vi "2014 Robot Global Data.vi"() -> ()   [LabVIEW 2013]
doc: "This global VI can contain as many global variables as you need. Place a control on the panel, give it a good name. To read or write to it from a VI, drag the icon to the diagram of that VI. You can also drag from the project. Click on the node to change which global you access. You shouldn't have multiple locations writing to a global or it will cause a race-condition."
uses:
  <vilib>/Rock Robotics/WPI/DriverStation/WPI_DriverStationRobotMode2.ctl
  <vilib>/Rock Robotics/WPI/Camera/WPI_CameraImageSize.ctl
panel:
  in  "Tab Control":T1(tab)=enum."I/O Definitions"
  in  "Enable Temp 16":bool
  in  "Enable Temp 15":bool
  in  "Enable Temp 14":bool
  in  "Enable Ejector":bool=TRUE
  in  "Enable Illuminators":bool
  in  "Enable PWM Wheels":bool
  in  "Enable CAN Voltage Wheels":bool=TRUE
  in  "Enable CAN Speed Wheels":bool
  in  "Enable Compressor":bool=TRUE
  in  "Enable Vision":bool
  in  "Enable I2C Accelerometer":bool=TRUE
  in  "Enable Gyro Temp":bool=TRUE
  in  "Enable Gyro":bool=TRUE
  in  "Enable Shooter Tilt":bool=TRUE
  in  "Enable Pickup Rollers":bool=TRUE
  in  "Enable Shooter Wheels":bool=TRUE
  in  "Robot Mode":T2=enum."Finish"
  in  "LED toggle rate (ms)":u32=250
  in  "image size":T3=enum."320x240"
  in  "Accelerometer Gain":dbl=1.0
  in  "Gyro Gain\n(VoltsPerDegree/Second)":dbl=0.007
  out "Gyro Temp":dbl
  out "Gyro Angle":dbl=2.5745306100192002
  out "Gyro Rate":dbl=-0.02367994921875
  out "Battery Voltage":dbl=12.69887799264
  out "X-Acceleration":i16
  out "Y-Acceleration":i16
  out "Z-Acceleration":i16
  in  "Drive Wheel Scale":dbl=1.0
  in  "Wheel Kd":dbl
  in  "Wheel Ki":dbl=0.004
  in  "Wheel Kp":dbl=0.5
  in  "RL_Wheel _Speed":dbl(slide)=6.053567521332485e-11 scale=-400.0..400.0
  in  "FL_Wheel_Speed":dbl(slide) scale=-400.0..400.0
  in  "RR_Wheel _Speed":dbl(slide) scale=-400.0..400.0
  in  "FR_Wheel_Speed":dbl(slide)=6.053567521332485e-11 scale=-400.0..400.0
  in  "Shooter Position 6":dbl=3.5
  in  "Shooter Position 5":dbl=3.0
  in  "Shooter Position 4":dbl=2.5
  in  "Shooter Position 3":dbl=2.0
  in  "Shooter Position 2":dbl=1.5
  in  "Shooter Position 1":dbl=1.0
  in  "Shooter Set Point":dbl=2.0
  in  "Shooter Lower Limit":dbl=0.05
  in  "Shooter Upper Limit":dbl=4.1
  out "Shooter Position":dbl(knob)=3.3318718420000004 scale=0.0..5.0
  in  "Pickup Roller Power":dbl(slide) scale=-1.0..1.0
  in  "Shooter Wheel Power":dbl(slide) scale=-1.0..1.0
  out "Button 12":bool
  out "Button 11":bool
  out "Button 10":bool
  out "Button 9":bool
  out "Button 8":bool
  out "Button 7":bool
  out "Button 6":bool
  out "Button 5":bool
  out "Button 4":bool
  out "Button 3":bool
  out "Button 2":bool
  out "Button 1":bool
  out "A-Axis":dbl=1.0
  out "Z-Axis":dbl
  out "Y-Axis":dbl=-0.007874015748031496
  out "X-Axis":dbl=-0.007874015748031496
  # "Sub-System Enablers"
  # "Preferences"
  # "Sensor Systems"
  # "Drive Wheel System"
  # "Shooter System"
  # "Joystick System"
  # "PWM OUTPUTS\nPWM 1 - Front Left Wheel (Optional)\nPWM 2 - Rear Left Wheel (Optional)\nPWM 3 - Front Right Wheel (Optional)\nPWM 4 - Rear Right Wheel (Optional)\nPWM 5 - Pick-Up Roller\nPWM 6 - Shooter Motor\nPWM 7 - \nPWM 8 - \nPWM 9 - \nPWM 10 - \n\nRELAY OUTPUTS\nRELAY 1 = Compressor\nRELAY 2 = \nRELAY 3 = \nRELAY 4 = \nRELAY 5 = \nRELAY 6 = \nRELAY 7 = \nRELAY 8 = \n\nSOLENOID OUTPUTS\nDO 1 = \nDO 2 = \nDO 3 = \nDO 4 = \nDO 5 = \nDO 6 = \nDO 7 = \nDO 8 =\n\nANALOG INPUTS\nAI 1 = Gyro\nAI 2 = Gyro Temperature\nAI 3 = Shooter Position\nAI 4 = \nAI 5 = \nAI 6 = \nAI 7 = \nAI 8 = Battery Voltage"
  # "DIGITAL I/O\nDIO 1 = Pressure Switch (Input)\nDIO 2 = Frisbee in Dustpan (Input) \nDIO 3 = Frisbee in Position 2 (Input)\nDIO 4 = Frisbee Leaving Shooter (Input)\nDIO 5 = Shooter Upper Limit (Input)\nDIO 6 = Shooter Lower Limit (Input)\nDIO 7 = \nDIO 8 = \nDIO 9 = \nDIO 10 = \nDIO 11 = \nDIO 12 = \nDIO 13 = \nDIO 14 = \n\nCAN BUS\nCAN 1 = Front Left Wheel (Max RPM = 400)\nCAN 2 = Rear Left Wheel (Max RPM = 400)\nCAN 3 = Front Right Wheel (Max RPM = 400)\nCAN 4 = Rear Right Wheel (Max RPM = 400)\nCAN 5 = Shooter Tilt\nCAN 6 = \nCAN 7 = \nCAN 8 = \n\nI2C ADDRESSES\n0x32 -> 0x33 = Accelerometer X Axis\n0x34 -> 0x35 = Accelerometer Y Axis\n0x36 -> 0x37 = Accelerometer Z Axis\n\nETHERNET ADDRESSES\n10.0.34.2 = cRIO\n10.0.34.3 = \n10.0.34.4 = \n10.0.34.5 = \n10.0.34.6 = \n10.0.34.7 = \n10.0.34.8 = \n10.0.34.9 = \n10.0.34.10 ="
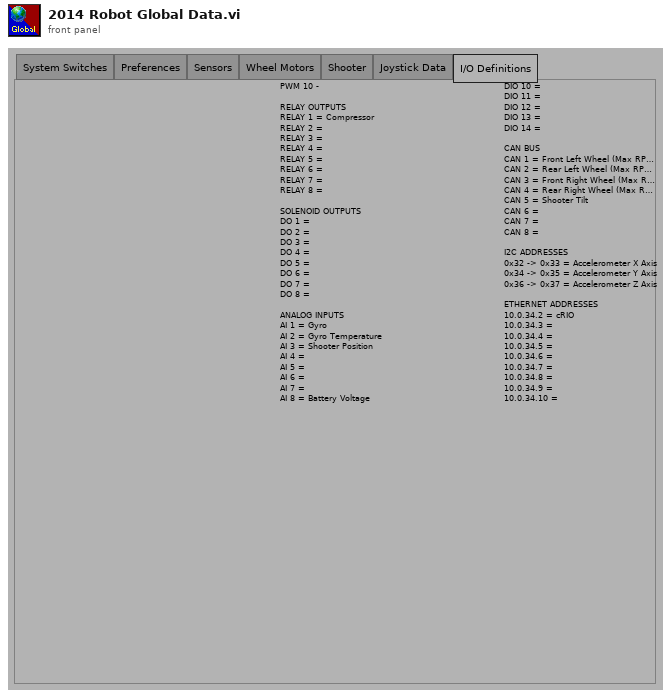
[diagram p1: front panel]
types:
  T1 = enum32{"System Switches", "Preferences", "Sensors", "Wheel Motors", "Shooter", "Joystick Data", "I/O Definitions"}
  T2 = typedef "WPI_DriverStationRobotMode2.ctl" = enum16{"Autonomous Disabled", "Autonomous Enabled", "Teleop Disabled", "Teleop Enabled", "Timeout", "Finish", "Test Disabled", "Test Enabled"}
  T3 = typedef "WPI_CameraImageSize.ctl" = enum16{"640x480", "320x240", "160x120"}
diagram:
